vi "Fill Maps.vi"(9 "Event Types":T2[](array[typedef]), 10 "Module names":string[](array[string]), 11 "DQMH Modules":refnum<vi>[](array[refnum])) -> (1 "Cancelled?":bool, 2 "map ref out":map{string, refnum<vi>}(c390), 3 "Tree Map out":T1)   [LabVIEW 2020, in "Panther Dashboard.lvlib"]
uses:
  Panther Dashboard.lvlib
  Event types--enum.ctl
  <vilib>/National Instruments/Tree Map/Tree Map Data.ctl
  <vilib>/National Instruments/Tree Map/Tree Map.lvlib
  <vilib>/ProgressBar/Progress Bar Dialog.lvclass
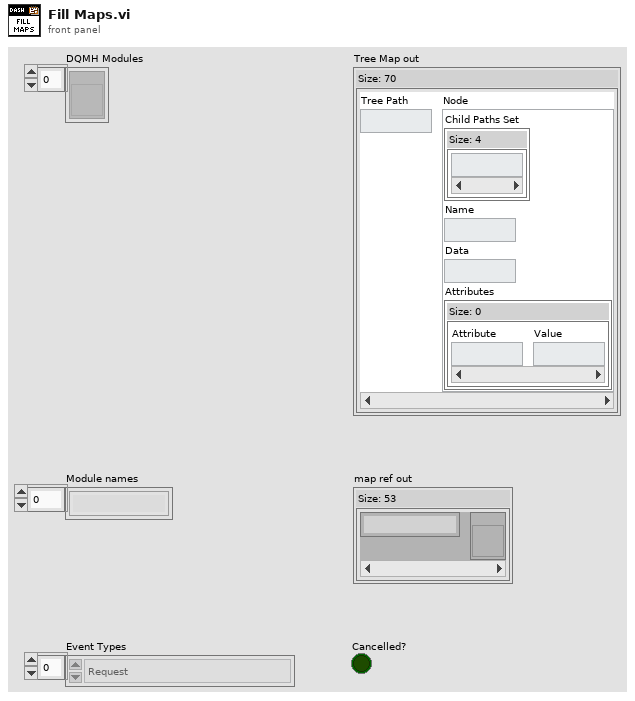
[diagram p1: front panel]
types:
  T1 = typedef "Tree Map.lvlib/Tree Map Data.ctl" = map{string, cluster{"Child Paths Set":set{string}, "Name":string, "Data":string, "Attributes":map{string, string}}}
  T2 = typedef "Panther Dashboard.lvlib/Event types--enum.ctl" = enum16{"Request", "Request and Wait for Reply", "Broadcast"}
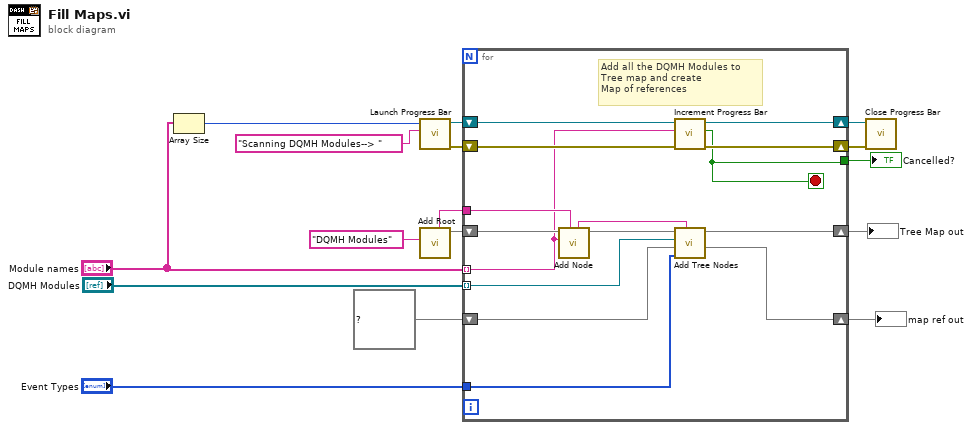
[diagram p0: block diagram]
diagram:
  n1 = Array Size(array="Module names") -> (size(s)=w5:i32)
  n2 = call <vilib>:"Launch Progress Bar.vi"("Main Title (\"Working...\")"="Scanning DQMH Modules--> " ("Main Title (\"Working...\")"), "Total Count"=w5) -> ("error out"=w16:errorcluster, "Progress Bar Dialog"=w8:refnum<class "Progress Bar Dialog.lvclass">)  [unwired: 8 in]
  n3 = call <vilib>:"Add Root.vi"("New Root Name"="DQMH Modules") -> ("Tree Map Out"=w10:T1, "Root Path"=w4:string)  [unwired: 9 in]
  n4 = for {
    shift-right: [w27] -> w12
    shift-left: w10 -> [w22]
    shift-right: [w29] -> w14
    shift-left: map{string, refnum<vi>} {} ("References Map") -> [w28]
    tunnel: "DQMH Modules" -> [w26] mode=indexing
    shift-right: [w24] -> w7
    shift-left: w8 -> [w25]
    shift-right: [w30] -> w15
    shift-left: w16 -> [w31]
    tunnel: w4 -> [w20]
    tunnel: "Event Types" -> [w23]
    tunnel: "Module names" -> [w18] mode=indexing
    tunnel: [w17] -> w1
    stop <- w17 stop-if-true
    # "Add all the DQMH Modules to\nTree map and create \nMap of references"
    n5 = call <vilib>:"Add Node.vi"("Parent Path"=w20, "New Node Name"=w18, "Tree Map In"=w22) -> ("Tree Map Out"=w21:T1, "New Node Path"=w19:string)  [unwired: 6 in, 1 out]
    n6 = call <vilib>:"Increment Progress Bar.vi"("error in (no error)"=w31, "Step Name (\"\")"=w18, "Progress Bar Dialog in"=w25) -> ("error out"=w30:errorcluster, "Cancelled?"=w17:bool, "Progress Bar Dialog out"=w24:refnum<class "Progress Bar Dialog.lvclass">)  [unwired: 6 in]
    n7 = call "Add Tree Nodes.vi"("Root path"=w19, "Event Types"=w23, "map ref in"=w28, "DQMH Lib In"=w26, "Tree Map in"=w21) -> ("map ref out"=w29:map{string, refnum<vi>}, "Tree Map out"=w27:T1)  [unwired: 5 in]
  }
  "map ref out" <- w14
  "Tree Map out" <- w12
  "Cancelled?" <- w1
  n8 = call <vilib>:"Close Progress Bar.vi"("error in (no error)"=w15, "Progress Bar Dialog"=w7) -> ()  [unwired: 9 in, 1 out]
